vi "Gateway_RecodeJson.vi"(8 "error in (no error)":errorcluster, 10 "Use Gateway to Monitor SSH traffic (recommended)":bool=TRUE, 11 "GatewayClass in":refnum<class "GatewayClass.lvclass">) -> (0 "error out":errorcluster, 2 "Re-coded MIDAS Reply":string, 3 "GatewayClass out":refnum<class "GatewayClass.lvclass">)   [LabVIEW 2018, in "feGEM Gateway.lvlib" / "GatewayClass.lvclass"]
uses:
  GatewayClass.lvclass
  GatewayClass.lvclass/GatewayClass.ctl
  <vilib>/regexp/Match Regular Expression.xnode
  DataPacker/Utilities/SSH_TUNNEL.lvclass
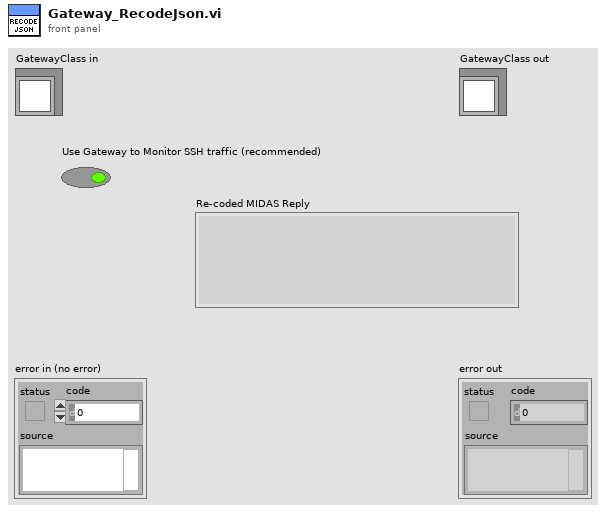
[diagram p1: front panel]
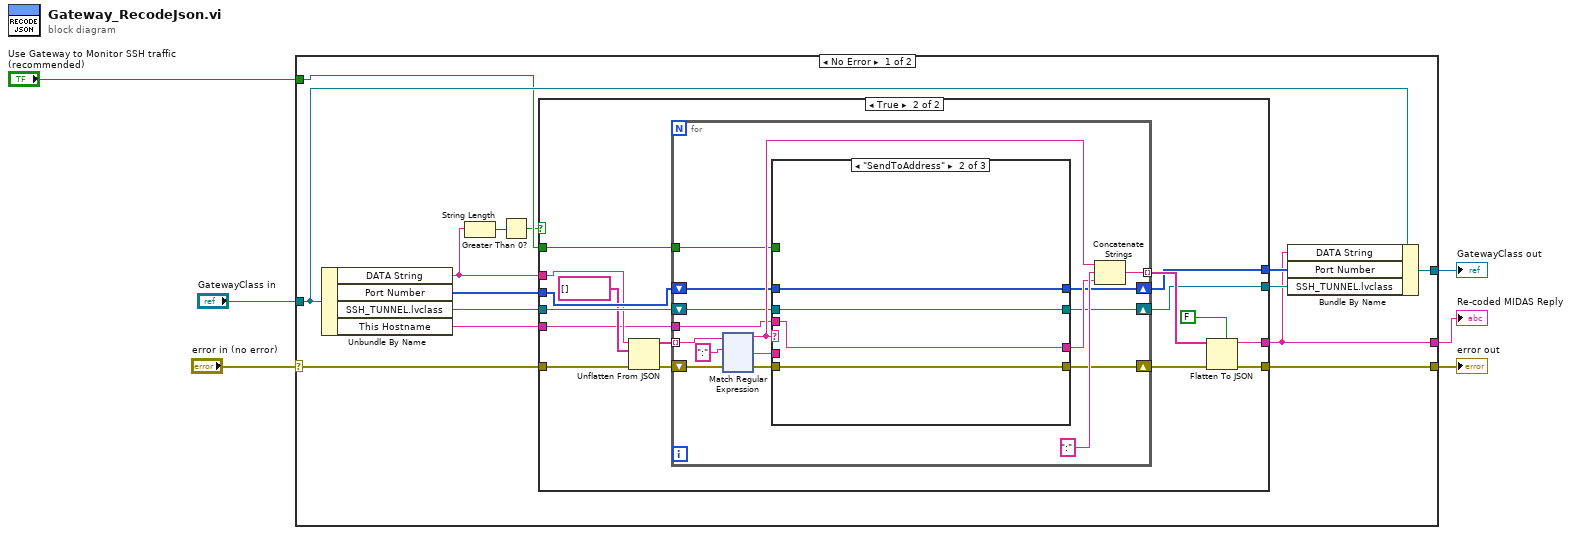
[diagram p0: block diagram]
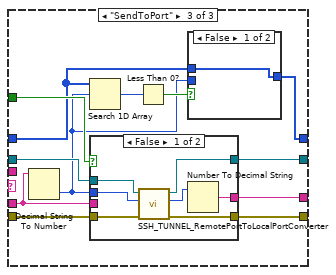
[diagram p4: hidden frame]
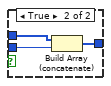
[diagram p5: hidden frame]
diagram:
  n1 = case shown="No Error" "error in (no error)" {
    selector: "error in (no error)" -> [w9 w206]
    tunnel: [w14 w206] -> w5
    tunnel: [w8 w205] -> w3
    tunnel: "GatewayClass in" -> [w19 w205]
    tunnel: "Use Gateway to Monitor SSH traffic (recommended)" -> [w17 _]
    tunnel: [w13 _] -> w1
    frame No Error {
      n2 = Unbundle By Name(w19) -> ("DATA String"=w12:string, "Port Number"=w20:u16[], "SSH_TUNNEL.lvclass"=w18:refnum<class "SSH_TUNNEL.lvclass">, "This Hostname"=w7:string)
      n3 = String Length(string=w12) -> (length=w11:i32)
      n4 = Greater Than 0?(x=w11) -> (x > 0?=w10:bool)
      n5 = case shown="True" w10 {
        tunnel: w20 -> [w24 w40]
        tunnel: w18 -> [w23 w36]
        tunnel: w17 -> [_ w35]
        tunnel: [w24 w34] -> w16
        tunnel: [w23 w33] -> w15
        tunnel: [w21 w32] -> w14
        tunnel: [w22 w31] -> w13
        tunnel: w12 -> [w22 w26]
        tunnel: w9 -> [w21 w27]
        tunnel: w7 -> [_ w25]
        frame False {
        }
        frame True {
          n6 = Unflatten From JSON(JSON string=w26, type and defaults=string[] [] ("Array"), error in (no error)=w27) -> (value=w29:string[], error out=w28:errorcluster)  [unwired: 4 in]
          n7 = for {
            tunnel: w29 -> [w56] mode=indexing
            shift-right: [w43] -> w39
            shift-left: w28 -> [w53]
            tunnel: [w49] -> w38 mode=indexing
            shift-right: [w47] -> w34
            shift-left: w40 -> [w48]
            shift-right: [w45] -> w33
            shift-left: w36 -> [w46]
            tunnel: w35 -> [w42]
            tunnel: w25 -> [w41]
            n8 = xnode "Match Regular Expression"("input string"=w56, "regular expression"=":", "error in"=w53) -> ("before match"=w52:string, "after match"=w54:string, "error out"=w44:errorcluster)  [unwired: 3 in, 2 out]
            n9 = case shown="\"SendToAddress\"" w52 {
              tunnel: w54 -> [w174 _ w184]
              tunnel: [w174 w178 w188] -> w50
              tunnel: w41 -> [_ w178 _]
              tunnel: w48 -> [w173 w177 w179]
              tunnel: [w173 w177 w180] -> w47
              tunnel: w46 -> [w171 w175 w190]
              tunnel: [w171 w175 w189] -> w45
              tunnel: w44 -> [w172 w176 w187]
              tunnel: [w172 w176 w186] -> w43
              tunnel: w42 -> [_ _ w185]
              frame "False", Default {
              }
              frame "SendToAddress" {
              }
              frame "SendToPort" {
                n10 = Decimal String To Number(string=w184) -> (number=w181:i32)  [unwired: 2 in, 1 out]
                n11 = Search 1D Array(1D array=w179, element=w181) -> (index of element=w183:i32)  [unwired: 1 in]
                n12 = case shown="False" w185 {
                  tunnel: w190 -> [w201 w204]
                  tunnel: [w200 w204] -> w189
                  tunnel: w181 -> [w199 _]
                  tunnel: [w197 w203] -> w188
                  tunnel: w187 -> [w196 w202]
                  tunnel: [w195 w202] -> w186
                  tunnel: w184 -> [_ w203]
                  frame False {
                    n13 = call "SSH_TUNNEL_RemotePortToLocalPortConverter.vi"("error in (no error)"=w196, "Remote Port Number"=w199, "SSH_TUNNEL in"=w201) -> ("error out"=w195:errorcluster, "Local Port Number"=w198:u16, "SSH_TUNNEL out"=w200:refnum<class "SSH_TUNNEL.lvclass">)  [unwired: 6 in]
                    n14 = Number To Decimal String(number=w198) -> (decimal integer string=w197:string)  [unwired: 1 in]
                  }
                  frame True {
                  }
                }
                n15 = Less Than 0?(x=w183) -> (x < 0?=w182:bool)
                n16 = case shown="False" w182 {
                  tunnel: w179 -> [w191 w194]
                  tunnel: w181 -> [_ w193]
                  tunnel: [w191 w192] -> w180
                  frame False {
                  }
                  frame True {
                    n17 = Build Array (concatenate)(w194, w193) -> (w192:i32[])
                  }
                }
              }
            }
            n18 = Concatenate Strings(w52, ":" ("string"), w50) -> (w49:string)
          }
          n19 = Flatten To JSON(enable LabVIEW extensions? (T)=FALSE, anything=w38, error in (no error)=w39) -> (JSON string=w31:string, 11:w32:errorcluster)
        }
      }
      n20 = Bundle By Name(cluster=w19, "DATA String"=w13, "Port Number"=w16, "SSH_TUNNEL.lvclass"=w15) -> (w8:refnum<class "GatewayClass.lvclass">)
    }
    frame Error {
    }
  }
  "error out" <- w5
  "GatewayClass out" <- w3
  "Re-coded MIDAS Reply" <- w1
